vi "serial open.vi"(1 "baud rate (9600)":u32=115200 caption="보 전송속도(9600)", 2 "Port":refnum<visa-resource-name>="COM4" caption="VISA 리소스 이름") -> (3 "에러 출력":errorcluster, 4 "연결된 문자열":string="VER\r", 5 "Version":string="VER 20081001-0000001-2-1\n\r")   [LabVIEW 2010]
uses:
  <vilib>/Instr/_visa.llb/VISA Flush IO Buffer Mask.ctl
  <vilib>/Instr/_visa.llb/VISA Configure Serial Port (Instr).vi
panel:
  out "Write data":u32=4
  out "Read Data":u32=26
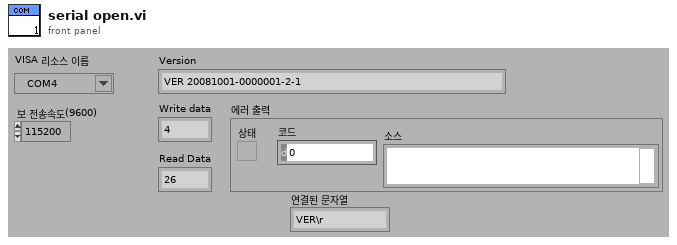
[diagram p1: front panel]
types:
  T1 = typedef "VISA Flush IO Buffer Mask.ctl" = u16
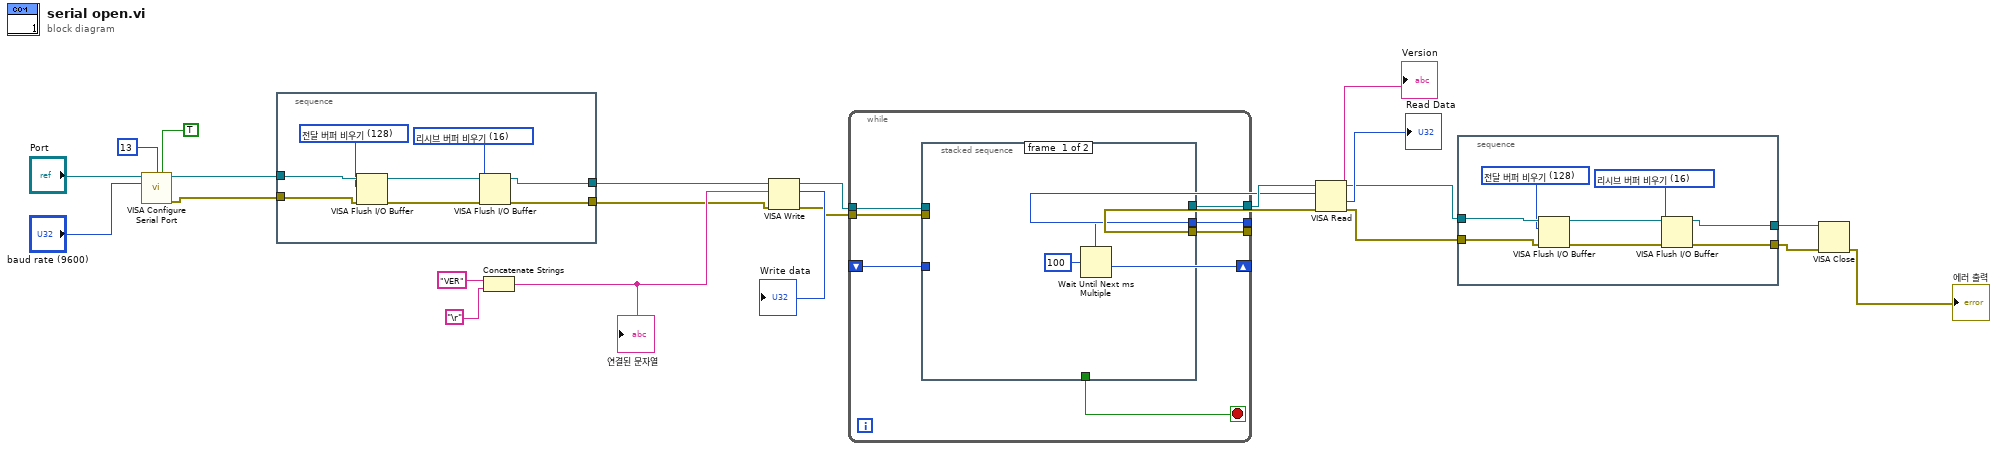
[diagram p0: block diagram]
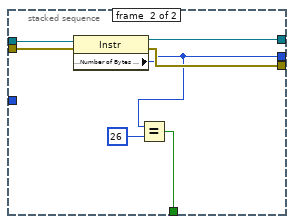
[diagram p2: hidden frame]
diagram:
  n1 = call-poly "VISA Configure Serial Port"("VISA resource name"="Port", "termination char\n(0xA = '\\n' = LF)"=i16 13 ("termination char\n(0xA = '\\n' = LF)"), "Enable Termination\nChar (T)"=TRUE ("Enable Termination\nChar (T)"), "baud rate (9600)"="baud rate (9600)") -> ("VISA resource name out"=w9:refnum<visa-resource-name>, "error out"=w8:errorcluster)  [unwired: 10 in]
  n2 = stacked-sequence {
    tunnel: w9 -> [w32]
    tunnel: w8 -> [w31]
    tunnel: [w27] -> w7
    tunnel: [w26] -> w6
    frame #0 {
      w25 = T1 16 items=["리시브 버퍼 비우기"=16, "전달 버퍼 디바이스에 쓰기"=32, "리시브 버퍼 비우기(I/O 없음)"=64, "전달 버퍼 비우기"=128] ("Mask")
      w30 = T1 128 items=["리시브 버퍼 비우기"=16, "전달 버퍼 디바이스에 쓰기"=32, "리시브 버퍼 비우기(I/O 없음)"=64, "전달 버퍼 비우기"=128] ("Mask")
      n3 = VISA Flush I/O Buffer(VISA resource name=w32, mask (16)=w30, error in (no error)=w31) -> (VISA resource name out=w29:refnum<visa-resource-name>, error out=w28:errorcluster)
      n4 = VISA Flush I/O Buffer(VISA resource name=w29, mask (16)=w25, error in (no error)=w28) -> (VISA resource name out=w27:refnum<visa-resource-name>, error out=w26:errorcluster)
    }
  }
  n5 = Concatenate Strings("VER" ("버퍼 쓰기"), "\r") -> (w14:string)
  "연결된 문자열" <- w14
  n6 = VISA Write(VISA resource name=w7, write buffer=w14, error in (no error)=w6) -> (VISA resource name out=w11:refnum<visa-resource-name>, return count=→"Write data":u32, error out=w10:errorcluster)
  n7 = while {
    tunnel: w11 -> [w39]
    tunnel: w10 -> [w38]
    tunnel: [w37] -> w21
    tunnel: [w36] -> w20
    tunnel: [w34] -> w19
    shift-right: [w34] -> _
    shift-left: _ -> [w33]
    stop <- w35 stop-if-true
    n8 = stacked-sequence {
      tunnel: w39 -> [_ w47]
      tunnel: w38 -> [_ w46]
      tunnel: [_ w45] -> w37
      tunnel: [_ w44] -> w36
      tunnel: [_ w43] -> w35
      tunnel: [_ w42] -> w34
      tunnel: w33 -> [_ _]
      frame #0 {
        n9 = Wait Until Next ms Multiple(millisecond multiple=u32 100 ("ms 배수")) -> ()  [unwired: 1 out]
      }
      frame #1 {
        n10 = property class="Instr"(reference=w47, error in=w46) -> (reference out=w44:refnum<visa-resource-name>, error out=w45:errorcluster, "Serial Settings:Number of Bytes at Serial Port"=w42:u32)
        n11 = Equal?(x=w42, y=u32 26) -> (x = y?=w43:bool)
      }
    }
  }
  n12 = VISA Read(VISA resource name=w20, byte count=w19, error in (no error)=w21) -> (VISA resource name out=w5:refnum<visa-resource-name>, read buffer=→"Version":string, return count=→"Read Data":u32, error out=w4:errorcluster)
  n13 = stacked-sequence {
    tunnel: w5 -> [w55]
    tunnel: w4 -> [w54]
    tunnel: [w50] -> w2
    tunnel: [w49] -> w3
    frame #0 {
      w48 = T1 16 items=["리시브 버퍼 비우기"=16, "전달 버퍼 디바이스에 쓰기"=32, "리시브 버퍼 비우기(I/O 없음)"=64, "전달 버퍼 비우기"=128] ("Mask")
      w53 = T1 128 items=["리시브 버퍼 비우기"=16, "전달 버퍼 디바이스에 쓰기"=32, "리시브 버퍼 비우기(I/O 없음)"=64, "전달 버퍼 비우기"=128] ("Mask")
      n14 = VISA Flush I/O Buffer(VISA resource name=w55, mask (16)=w53, error in (no error)=w54) -> (VISA resource name out=w52:refnum<visa-resource-name>, error out=w51:errorcluster)
      n15 = VISA Flush I/O Buffer(VISA resource name=w52, mask (16)=w48, error in (no error)=w51) -> (VISA resource name out=w50:refnum<visa-resource-name>, error out=w49:errorcluster)
    }
  }
  n16 = VISA Close(VISA resource name=w2, error in (no error)=w3) -> (error out=→"에러 출력":errorcluster)
